vi "Is Library SourceOnly.vi"(8 "error in":errorcluster, 9 "Library Ref in":refnum<vi>, 10 "Library Path":path) -> (0 "error out":errorcluster, 1 "Library Ref out":refnum<vi>, 2 "Is SourceOnly?":bool)   [LabVIEW 2020]
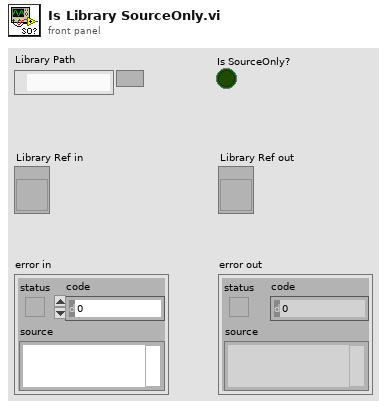
[diagram p1: front panel]
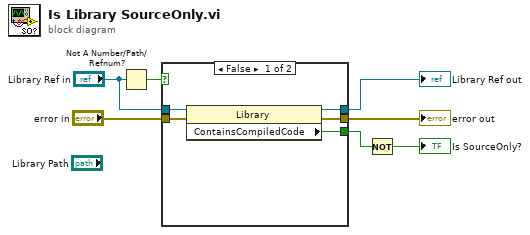
[diagram p0: block diagram]
diagram:
  n1 = Not A Number/Path/Refnum?(number/path/refnum="Library Ref in") -> (NaN/Path/Refnum?=w1:bool)
  n2 = case shown="False" w1 {
    tunnel: "error in" -> [w12 w14]
    tunnel: [w11 w14] -> w6
    tunnel: [w10 _] -> w4
    tunnel: [w9 w13] -> w3
    tunnel: "Library Ref in" -> [w8 w13]
    frame False {
      n3 = property class="Library"(reference=w8, error in=w12) -> (reference out=w9:refnum<vi>, error out=w11:errorcluster, "ContainsCompiledCode"=w10:bool)
    }
    frame True {
      # "Placeholder."
    }
  }
  "error out" <- w6
  "Library Ref out" <- w3
  n4 = Not(x=w4) -> (.not. x?=→"Is SourceOnly?":bool)
